vi "Construct Digital Trigger Names.vi"(8 "error in":errorcluster, 11 "4300 in":refnum<class "4300.lvclass">) -> (0 "error out":errorcluster, 3 "4300 out":refnum<class "4300.lvclass">)   [LabVIEW 2019, in "4300.lvlib" / "4300.lvclass"]
uses:
  Library/4300.lvclass
  C:/Users/Public/Documents/Development/builds/Instruments/AnalogInput.lvlibp/Library/AnalogInput.lvclass
  Library/4300.lvclass/4300.ctl
  builds/Instruments/AnalogInput.lvlibp/Accessors/Triggering/Read Enable Digital Trigger.vi
  <resource>/objmgr/daqmx.rc
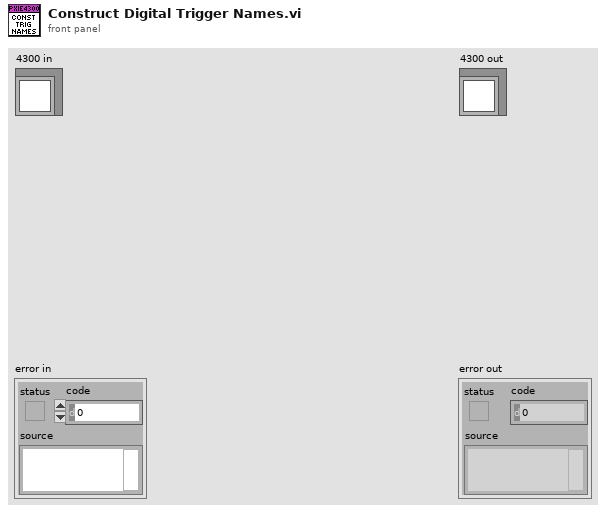
[diagram p1: front panel]
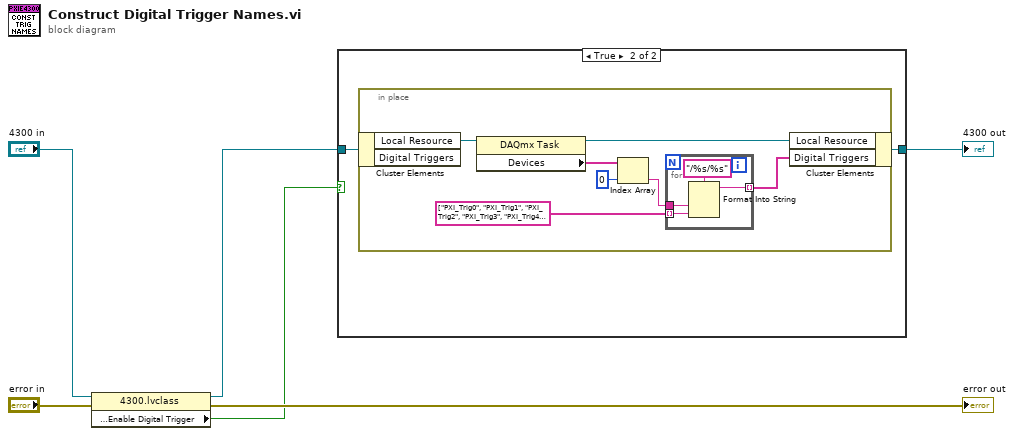
[diagram p0: block diagram]
diagram:
  n1 = property class="4300.lvclass"(reference="4300 in", error in="error in") -> (reference out=w2:refnum<class "4300.lvclass">, error out=→"error out":errorcluster, "Accessors:Config:Enable Digital Trigger"=w1:bool)
  n2 = case shown="True" w1 {
    tunnel: [w7 w9] -> w5
    tunnel: w2 -> [w7 w8]
    frame False {
    }
    frame True {
      n3 = in-place {
        n4 = in-place-cluster #1(w8) -> ("Local Resource"=w16:refnum<k21>)  [unwired: 1 out]
        n5 = property class="DAQmx Task"(reference=w16) -> (reference out=w15:refnum<k21>, "Devices"=w14:tag[])  [unwired: 1 in, 1 out]
        n6 = Index Array(array=w14, index=0) -> (element=w11:tag)
        n7 = for {
          tunnel: w11 -> [w20]
          tunnel: [w18] -> w10 mode=indexing
          tunnel: string[] ["PXI_Trig0", "PXI_Trig1", "PXI_Trig2", "PXI_Trig3", "PXI_Trig4", "PXI_Trig5", "PXI_Trig6", "PXI_Trig7"] ("Array 2") -> [w17] mode=indexing
          n8 = Format Into String(format string="/%s/%s", w20, w17) -> (resulting string=w18:string)  [unwired: 2 in, 1 out]
        }
        n9 = in-place-cluster #1("Local Resource"=w15, "Digital Triggers"=w10) -> (w9:refnum<class "4300.lvclass">)
      }
    }
  }
  "4300 out" <- w5
